vi "Read AzPA.vi"(8 "error in (no error)":errorcluster, 11 "ObjectPA in":refnum<class "ObjectPA.lvclass">) -> (0 "error out":errorcluster, 2 "AzPA":dbl[unit]=5.817764173314432e-05, 3 "ObjectPA out":refnum<class "ObjectPA.lvclass">)   [LabVIEW 2014, in "TCSDataDefinitions.lvlib" / "TCSPublicStatus.lvlib" / "PointingPositions.lvlib" / "ObjectPA.lvclass"]
uses:
  ObjectPA.lvclass
  ObjectPA.lvclass/ObjectPA.ctl
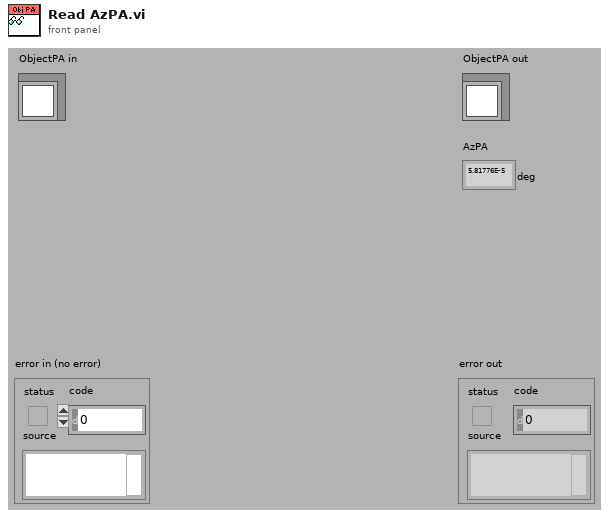
[diagram p1: front panel]
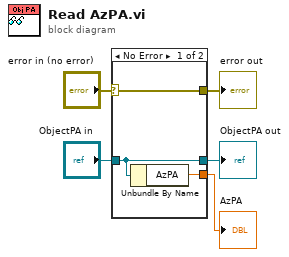
[diagram p0: block diagram]
diagram:
  n1 = case shown="No Error" "error in (no error)" {
    selector: "error in (no error)" -> [w8 w9]
    tunnel: [w8 w9] -> w4
    tunnel: [w7 w10] -> w2
    tunnel: "ObjectPA in" -> [w7 w10]
    tunnel: [w6 _] -> w1
    frame No Error {
      n2 = Unbundle By Name(w7) -> ("AzPA"=w6:dbl[unit])
    }
    frame Error {
    }
  }
  "error out" <- w4
  "ObjectPA out" <- w2
  "AzPA" <- w1
